vi "PowerControlDlg.vi"(3 "电源频率(Hz)":string="1", 8 "error out":errorcluster caption="error in") -> (0 "error out":errorcluster, 1 "倍数":string, 2 "NY":bool, 4 "电源电压(V)out":string="1", 5 "电压系数out":string="10")   [LabVIEW 2014, in "PowerControl.lvlib"]
uses:
  PowerControl.lvlib
  Acquisition/HW Configuration.ctl
  DataBase/DataBase.lvlib
  DetectElecrodes/DetectElectros.lvlib
  Acquisition/Acquisitions.lvlib
panel:
  out "电流值":dbl
  in  "电流系数":string="10"
  in  "电压系数":string="0.01"
  in  "备注":string
  in  "退出":bool
  in  "退出按钮":bool
  in  "确定按钮":bool
  in  "电源电压(V)":string="1"
  # "（1V~5V）"
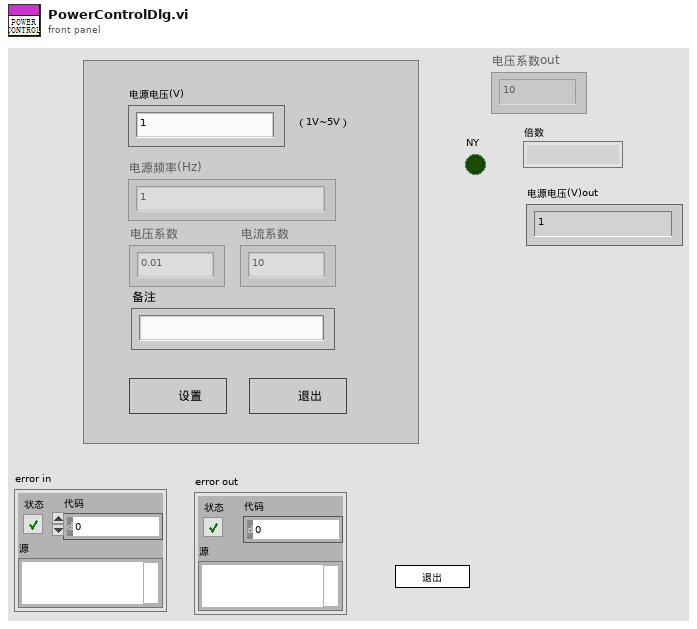
[diagram p1: front panel]
types:
  T1 = enum32{"invalid app kind", "Development System", "Run Time System", "Student Edition", "Embedded LabVIEW", "Evaluation", "Custom"}
  T2 = enum8{"Enabled", "Disabled", "Disabled and Grayed Out"}
  T3 = enum32{"Invalid", "Standard", "Closed", "Hidden", "Minimized", "Maximized"}
  T4 = typedef "Acquisitions.lvlib/HW Configuration.ctl" = cluster{"Physical Channel":tag, "Maximum Input":dbl, "Minimum Input":dbl, "Sample Rate":dbl, "Number of Samples":i32}
  T5 = cluster{"Core":cluster{"Current VI Reference":refnum<vi>, "Close Panel on Exit?":bool}, "Your Boolean data":bool, "Your string data":string, "V值":dbl, "倍数":string, "实际V值":string}
  T6 = cluster{"Current VI Reference":refnum<vi>, "Close Panel on Exit?":bool}
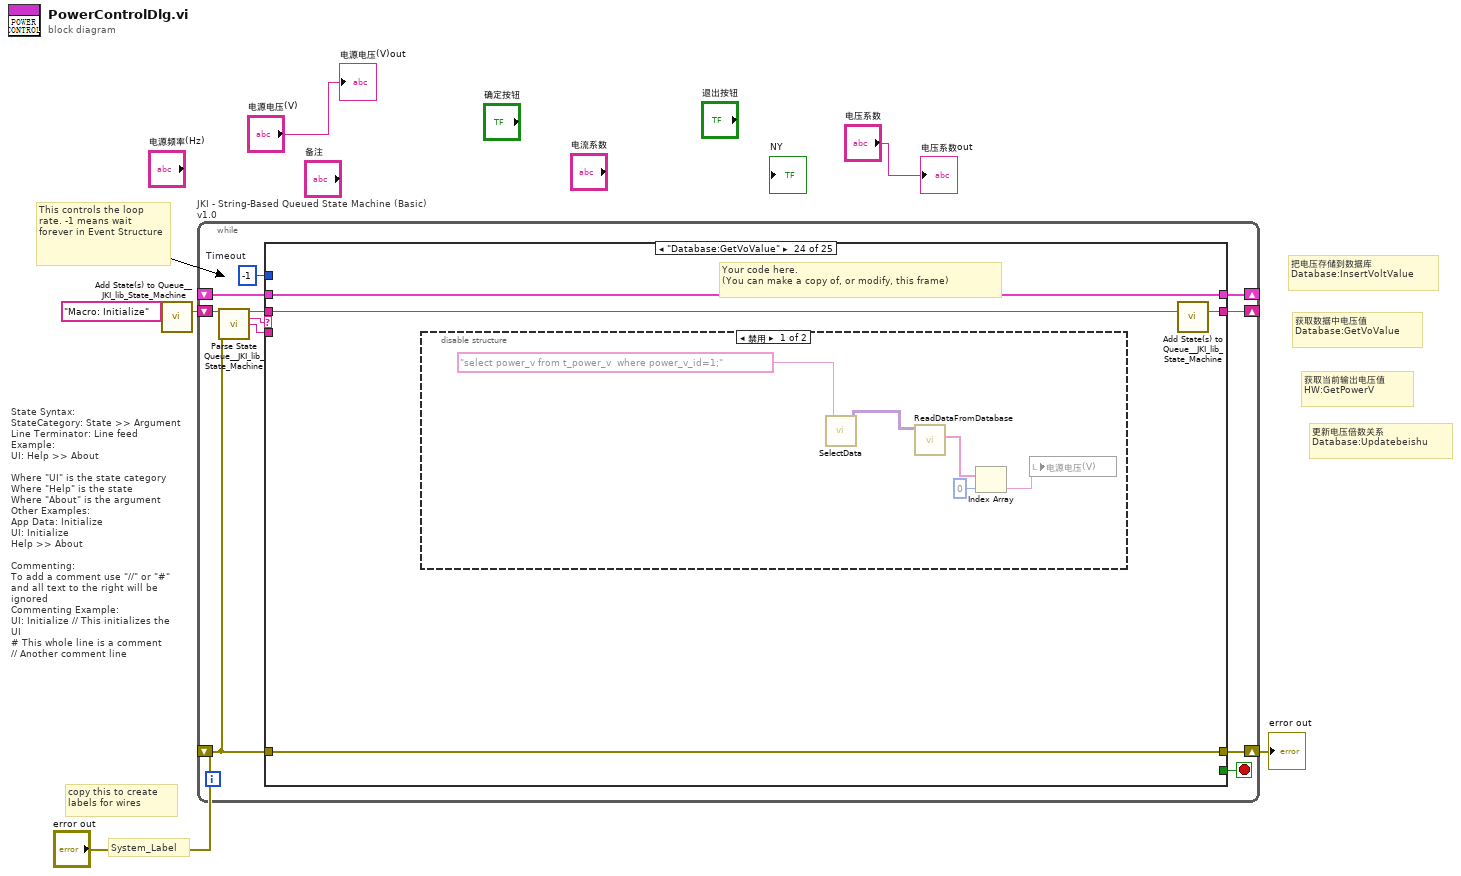
[diagram p0: block diagram]
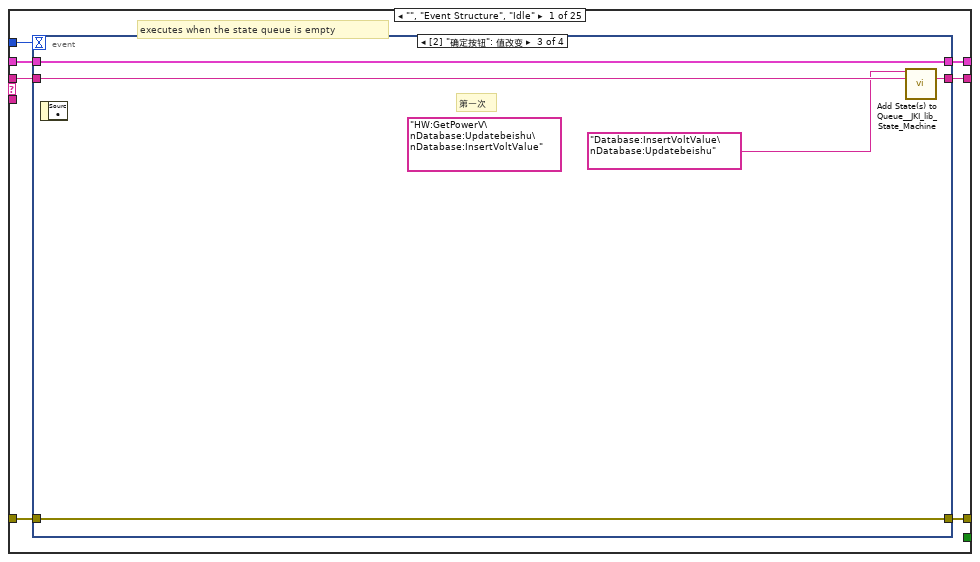
[diagram p2: hidden frame]
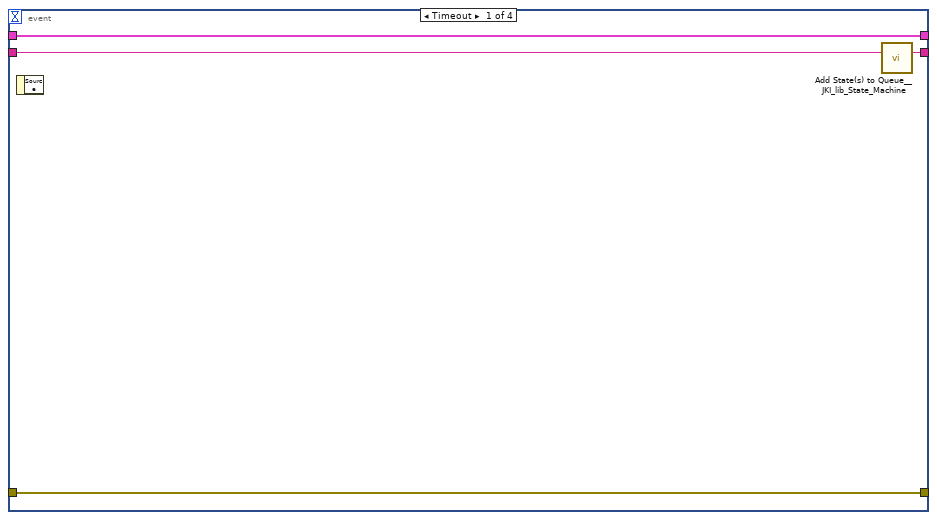
[diagram p3: hidden frame]
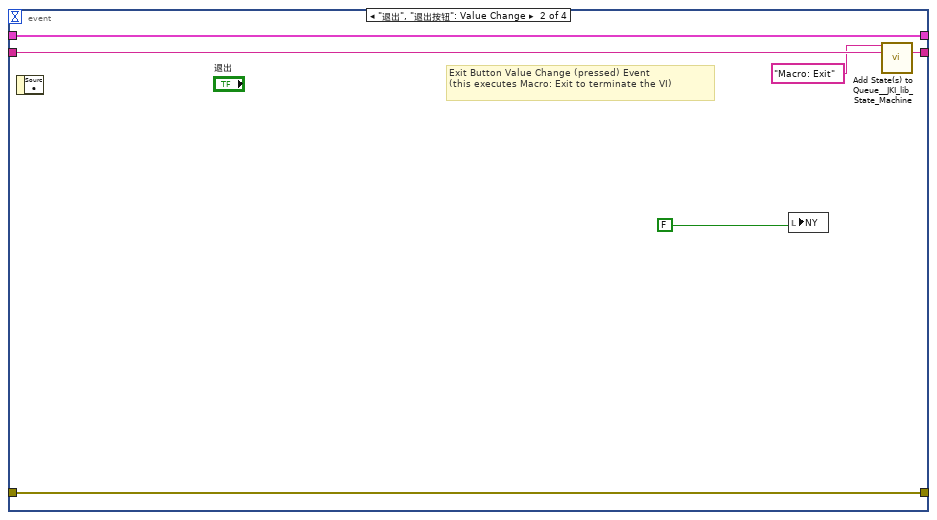
[diagram p4: hidden frame]
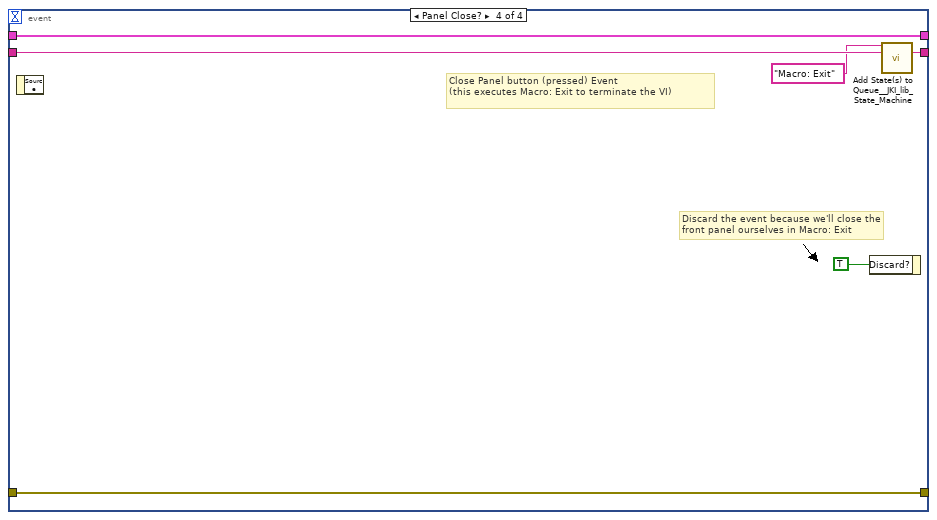
[diagram p5: hidden frame]
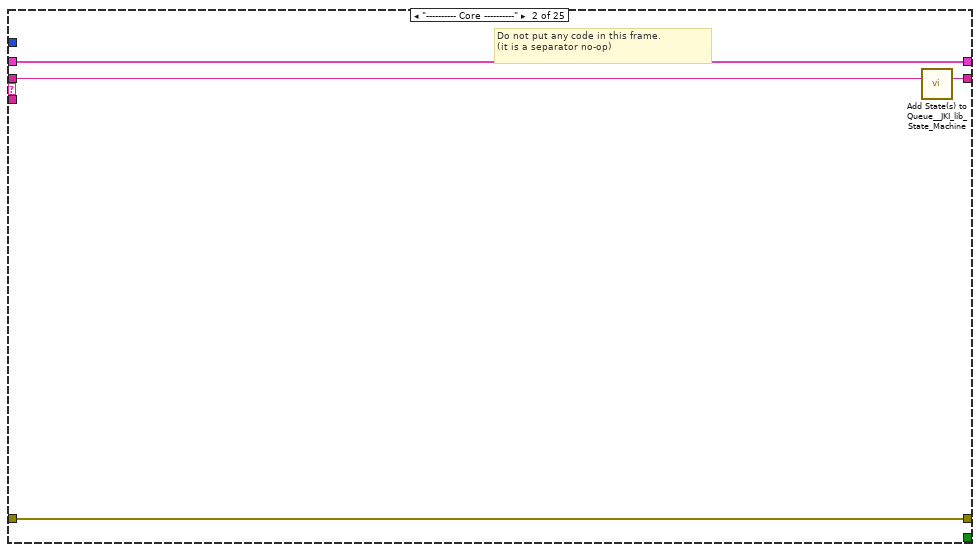
[diagram p6: hidden frame]
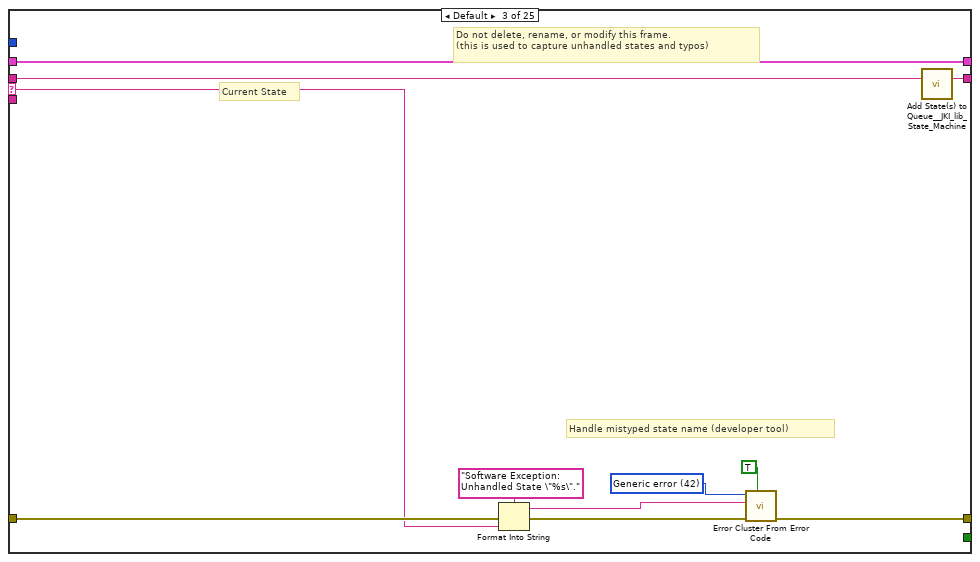
[diagram p7: hidden frame]
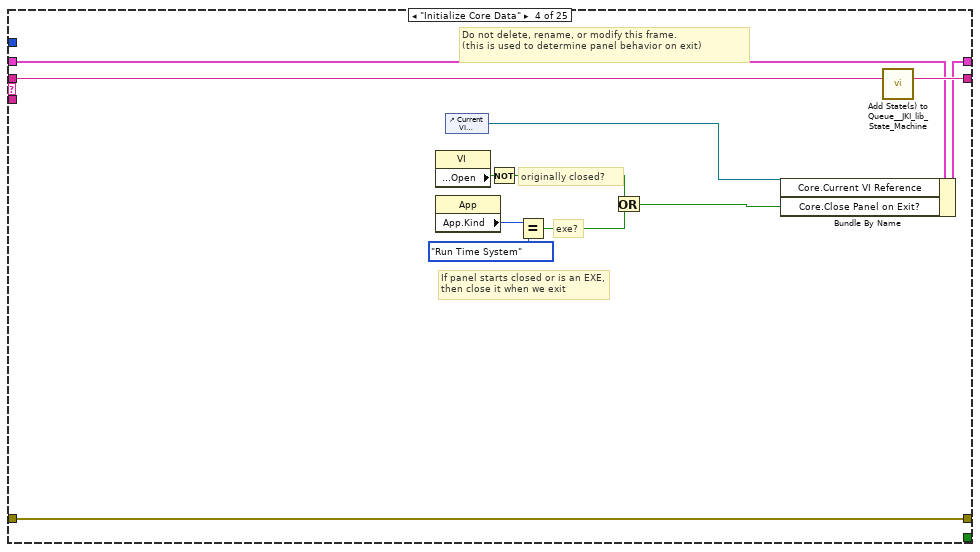
[diagram p8: hidden frame]
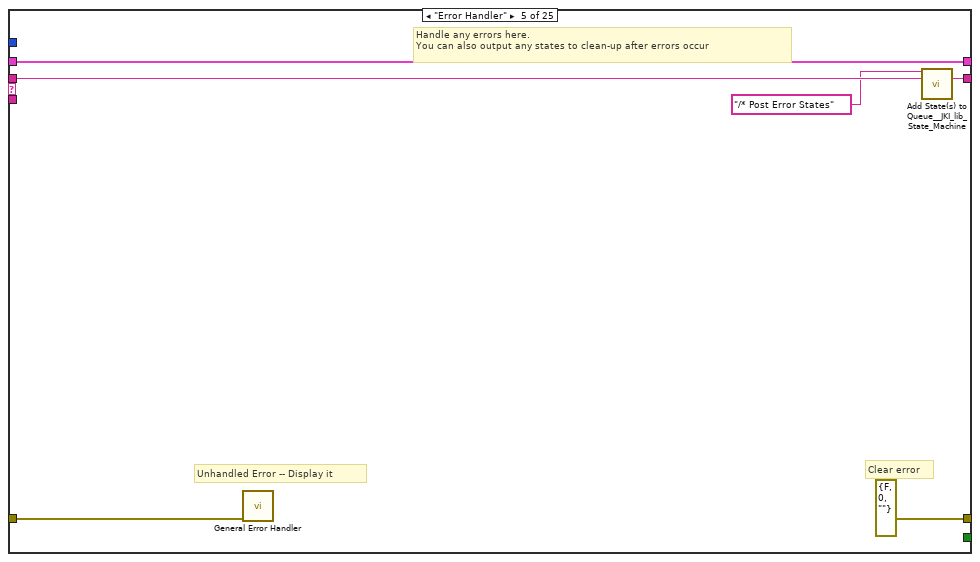
[diagram p9: hidden frame]
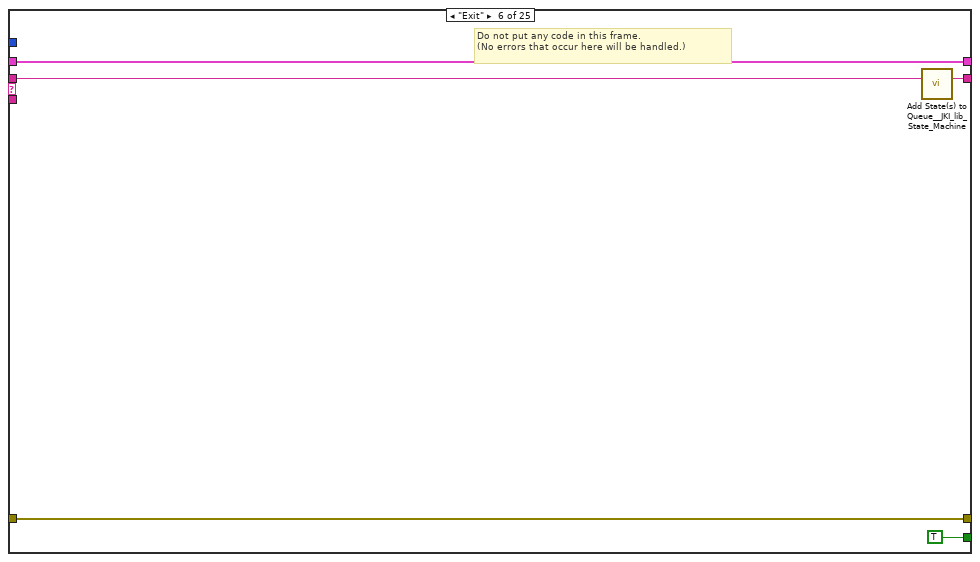
[diagram p10: hidden frame]
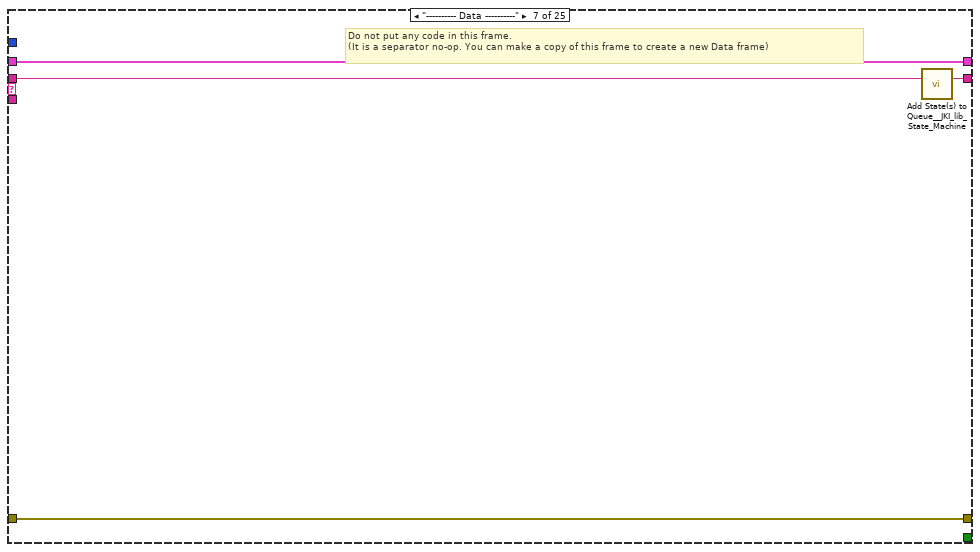
[diagram p11: hidden frame]
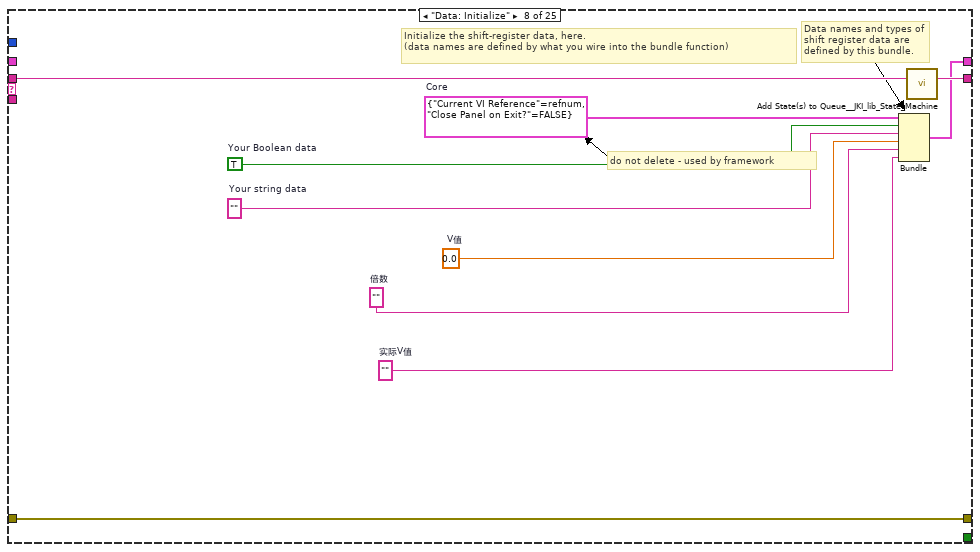
[diagram p12: hidden frame]
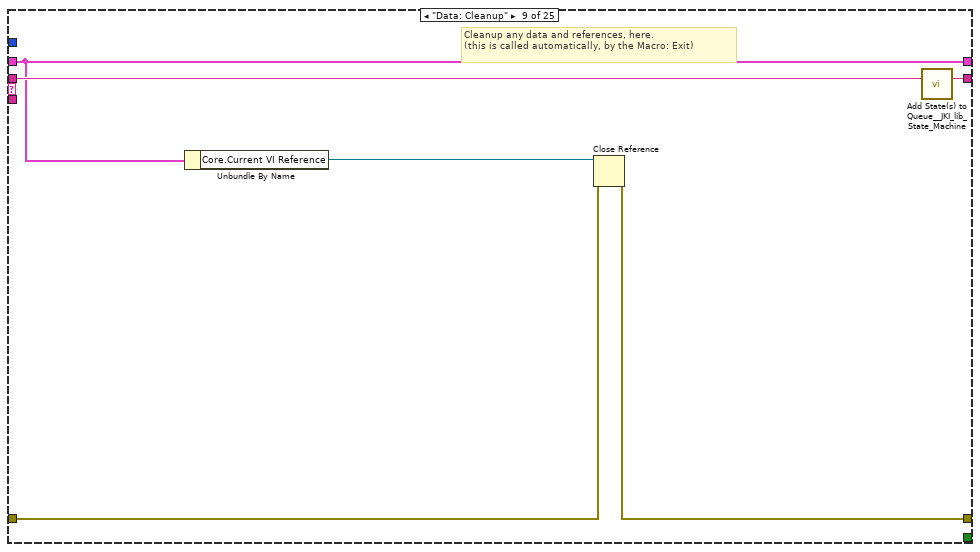
[diagram p13: hidden frame]
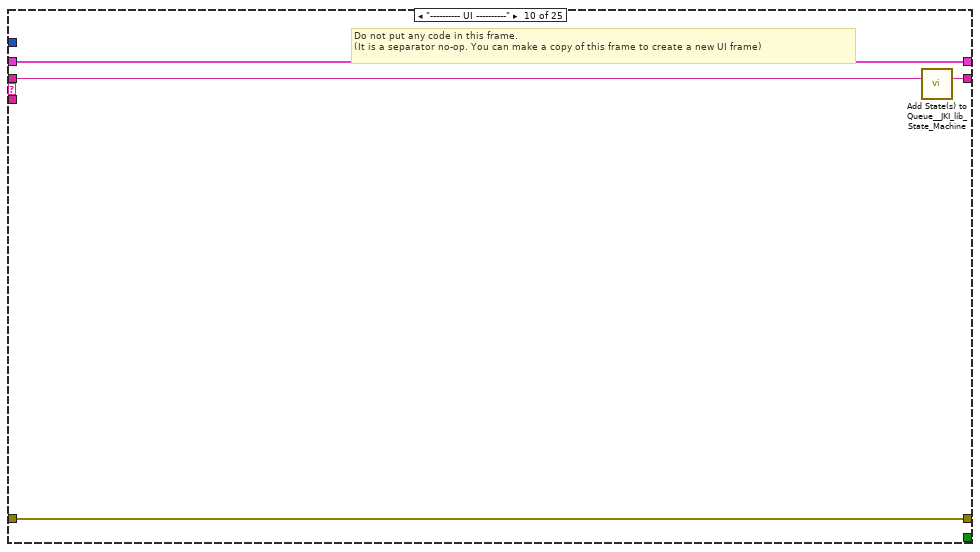
[diagram p14: hidden frame]
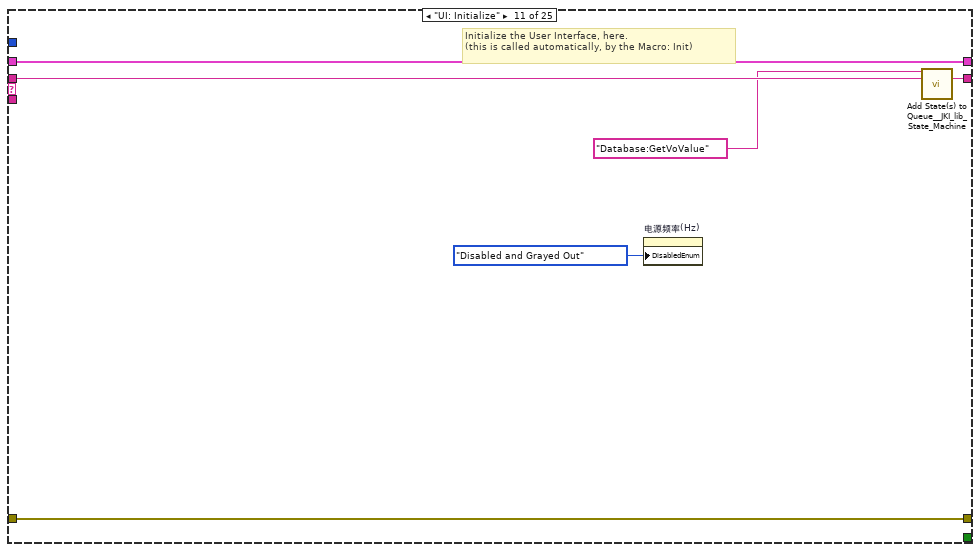
[diagram p15: hidden frame]
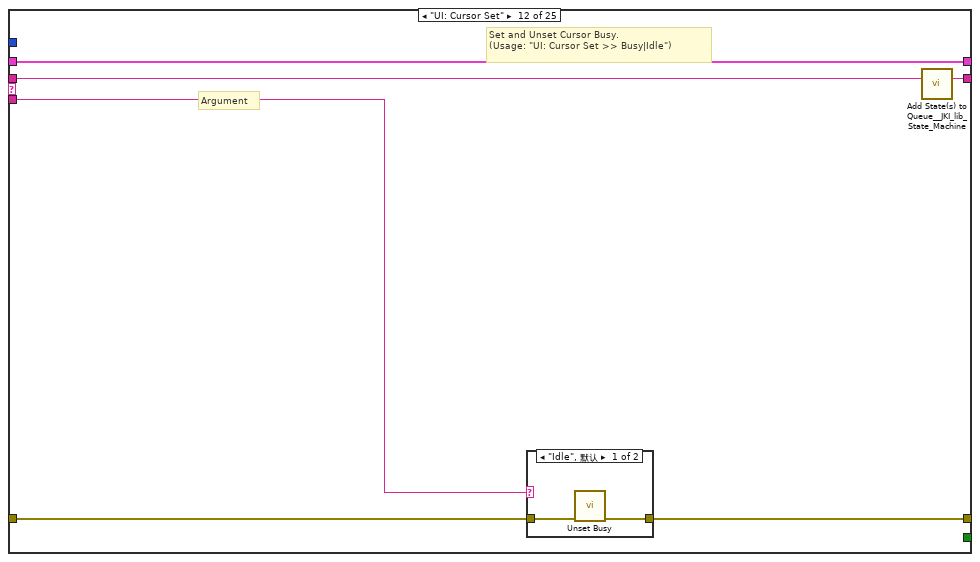
[diagram p16: hidden frame]
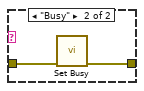
[diagram p17: hidden frame]
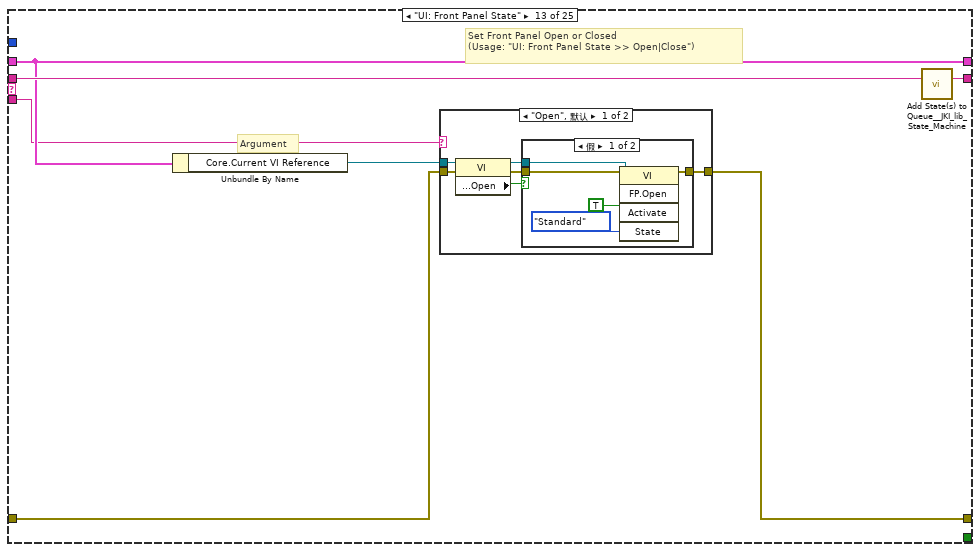
[diagram p18: hidden frame]
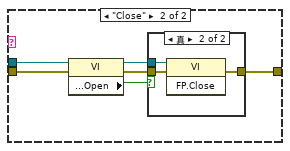
[diagram p20: hidden frame]
diagram:
  # "更新电压倍数关系\nDatabase:Updatebeishu"
  # "获取当前输出电压值\nHW:GetPowerV"
  # "获取数据中电压值\nDatabase:GetVoValue"
  # "把电压存储到数据库\nDatabase:InsertVoltValue"
  # "State Syntax:\nStateCategory: State >> Argument\nLine Terminator: Line feed\nExample:\nUI: Help >> About\n\nWhere \"UI\" is the state category\nWhere \"Help\" is the state\nWhere \"About\" is the argument\nOther Examples:\nApp Data: Initialize\nUI: Initialize\nHelp >> About\n\nCommenting:\nTo add a comment use \"//\" or \"#\" and all text to the right will be ignored\nCommenting Example:\nUI: Initialize // This initializes the UI\n# This whole line is a comment\n// Another comment line"
  # "copy this to create labels for wires"
  # "This controls the loop rate. -1 means wait forever in Event Structure"
  # "System_Label"
  n1 = call <vilib>:"Add State(s) to Queue__JKI_lib_State_Machine.vi"("State(s) in (\"\")"="Macro: Initialize") -> ("States Out"=w6:string)  [unwired: 14 in]
  n2 = while "JKI - String-Based Queued State Machine (Basic) v1.0" {
    shift-right: [w10] -> _
    shift-left: _ -> [w9]
    shift-right: [w13] -> w3
    shift-left: "error out" -> [w7]
    shift-right: [w12] -> _
    shift-left: w6 -> [w14]
    stop <- w11 stop-if-true
    w8 = -1  # Timeout
    n3 = call <vilib>:"Parse State Queue__JKI_lib_State_Machine.vi"("State Queue"=w14, "Error In (no error)"=w7) -> ("Remaining States"=w16:string, "Current State"=w17:string, "Arguments"=w15:string)  [unwired: 11 in]
    n4 = case shown="\"Database:GetVoValue\"" w17 {
      selector: w17 -> [_ _ w50 _ _ _ _ _ _ _ _ _ _ _ _ _ _ _ _ _ _ _ _ _ _]
      tunnel: w16 -> [w24 w49 w54 w72 w78 w83 w87 w97 w103 w107 w113 w119 w130 w156 w161 w171 w175 w179 w183 w187 w212 w216 w224 w239 w253]
      tunnel: w15 -> [_ _ _ _ _ _ _ _ _ _ _ w114 w124 _ _ _ _ _ _ _ _ _ _ _ _]
      tunnel: w9 -> [w22 w46 w52 w63 w75 w81 w84 _ w98 w104 w111 w117 w126 w153 w158 w168 w172 w176 w180 w184 w209 w213 w221 w236 w250]
      tunnel: [w21 w47 w56 w69 errorcluster {"status"=FALSE, "code"=0, "source"=""} ("error out") w80 w85 w94 w99 w105 w110 w115 w127 w154 w159 w169 w173 w177 w181 w185 w210 w214 w222 w237 w251] -> w13
      tunnel: w7 -> [w20 w47 w55 w69 w74 w80 w85 w94 w100 w105 w110 w116 w128 w154 w159 w169 w173 w177 w181 w185 w210 w214 w222 w237 w251]
      tunnel: [w23 w48 w53 w71 w77 w82 w86 w96 w102 w106 w112 w118 w129 w155 w160 w170 w174 w178 w182 w186 w211 w215 w223 w238 w252] -> w12
      tunnel: [_ _ _ _ _ TRUE _ _ _ _ _ _ _ _ _ _ _ _ _ _ _ _ _ _ _] -> w11
      tunnel: [w19 w46 w52 w70 w75 w81 w84 w95 w98 w104 w111 w117 w126 w153 w158 w168 w172 w176 w180 w184 w208 w213 w221 w236 w250] -> w10
      tunnel: w8 -> [w18 _ _ _ _ _ _ _ _ _ _ _ _ _ _ _ _ _ _ _ _ _ _ _ _]
      frame "", "Event Structure", "Idle" {
        # "executes when the state queue is empty"
        n5 = event shown="[2] \"确定按钮\": 值改变" {
          selector: _ -> [_ _ _ _]
          dyn-events: _ -> [_ _ _ _]
          timeout: w18 -> [_ _ _ _]
          tunnel: w24 -> [w28 w34 w39 w45]
          tunnel: [w27 w33 w38 w44] -> w23
          tunnel: w22 -> [w25 w31 w36 w42]
          tunnel: [w26 w32 w37 w43] -> w21
          tunnel: w20 -> [w26 w32 w37 w43]
          tunnel: [w25 w31 w36 w42] -> w19
          event Timeout {
            n6 = event-data() -> ()  [unwired: 1 in, 1 out]
            n7 = call <vilib>:"Add State(s) to Queue__JKI_lib_State_Machine.vi"("State(s) in (\"\")"=w28) -> ("States Out"=w27:string)  [unwired: 14 in]
          }
          event "退出", "退出按钮": Value Change {
            # "Exit Button Value Change (pressed) Event\n(this executes Macro: Exit to terminate the VI)"
            n8 = event-data() -> ()  [unwired: 1 in, 1 out]
            n9 = local write "NY"(FALSE) -> ()
            n10 = call <vilib>:"Add State(s) to Queue__JKI_lib_State_Machine.vi"("State(s) in Front (\"\")"="Macro: Exit", "State(s) in (\"\")"=w34) -> ("States Out"=w33:string)  [unwired: 13 in]
          }
          event "确定按钮": Value Change {
            (unwired) "HW:GetPowerV\nDatabase:Updatebeishu\nDatabase:InsertVoltValue"
            # "第一次"
            n11 = event-data() -> ()  [unwired: 1 in, 1 out]
            n12 = call <vilib>:"Add State(s) to Queue__JKI_lib_State_Machine.vi"("State(s) in Front (\"\")"="Database:InsertVoltValue\nDatabase:Updatebeishu", "State(s) in (\"\")"=w39) -> ("States Out"=w38:string)  [unwired: 13 in]
          }
          event Panel Close? {
            # "Discard the event because we'll close the front panel ourselves in Macro: Exit"
            # "Close Panel button (pressed) Event\n(this executes Macro: Exit to terminate the VI)"
            n13 = event-data() -> ()  [unwired: 1 in, 1 out]
            n14 = event-data("Discard?"=TRUE) -> ()  [unwired: 1 in, 1 out]
            n15 = call <vilib>:"Add State(s) to Queue__JKI_lib_State_Machine.vi"("State(s) in Front (\"\")"="Macro: Exit", "State(s) in (\"\")"=w45) -> ("States Out"=w44:string)  [unwired: 13 in]
          }
        }
      }
      frame "---------- Core ----------" {
        # "Do not put any code in this frame.\n(it is a separator no-op)"
        n16 = call <vilib>:"Add State(s) to Queue__JKI_lib_State_Machine.vi"("State(s) in (\"\")"=w49) -> ("States Out"=w48:string)  [unwired: 14 in]
      }
      frame Default {
        w59 = 42 items=["No error", "Argument error", "Memory is full", "Out of zone", "End of file", "File already open", "Generic file I/O error", "File not found", "File permission error", "Disk is full", "Duplicate path", "Too many files open", "System feature not enabled", "Resource file not found", "Cannot add resource", "Resource not found", "Image not found", "Image memory error", "Pen does not exist", "Config type invalid", "Config token not found", "Config parse error", "Config memory error", "Bad external code format", "Bad external code offset", "External code not present", "Null window", "Destroy window error", "Null menu", "Print aborted", "Bad print record", "Print driver error", "Windows error during printing", "Memory error during printing", "Print dialog error", "Generic print error", "Invalid device refnum", "Device not found", "Device parameter error", "Device unit error", "Cannot open device", "Device call aborted", "Generic error", "Cancelled by user", "Object ID too low", "Object ID too high", "Object not in heap", "Unknown heap", "Unknown object (invalid DefProc)", "Unknown object (DefProc not in table)", "Message out of range", "Invalid (null) method", "Unknown message", "Manager call not supported", "Bad address", "Network operation in progress", "Network operation timed out", "Connection is busy", "Network attribute not supported", "Network error", "Address in use", "System out of memory", "Connection aborted", "Connection refused", "Not connected", "Already connected", "Connection closed", "Initialization error (interapplication manager)", "Bad occurrence", "Wait on unbound occurrence handler", "Occurrence queue overflow", "Datalog type conflict", "Unused", "Unrecognized type (interapplication manager)", "Memory corrupt", "Failed to make temporary DLL", "Old CIN version", "Drag socket not found", "Failed to load drop-object", "Failed to register OLE object", "Failed to release OLE object", "Format specifier type mismatch", "Unknown format specifier", "Too few format specifiers", "Too many format specifiers", "Scan failed", "Newer CIN version", "Error converting to variant", "Runtime menu error", "Password tampered", "Variant attribute not found", "Incompatible variant data type", "Event data is not available", "Event Store is not present", "Occurrence is not found", "Event Queue is not created", "Event info is not available", "Refnum passed is NULL", "Error retrieving Class GUID", "Error retrieving CoClass GUID", "Error retrieving TypeLib GUID.", "Bad built application magic bytes.", "Specific driver is different from the specific driver associated with the Logical Name.", "There is no session opened to the class driver.", "Max Error", "MAX - Error with config objects", "MAX - Error loading configuration", "MAX - Group not supported"]
        # "Current State"
        # "Do not delete, rename, or modify this frame.\n(this is used to capture unhandled states and typos)"
        # "Handle mistyped state name (developer tool)"
        n17 = Format Into String(format string="Software Exception: Unhandled State \"%s\"." ("message"), error in=w55, w50) -> (resulting string=w58:string, error out=w57:errorcluster)  [unwired: 1 in]
        n18 = call <vilib>:"Error Cluster From Error Code.vi"("show call chain? (False)"=TRUE, "error in (no error)"=w57, "error message (\"\")"=w58, "error code (0)"=w59) -> ("error out"=w56:errorcluster)  [unwired: 5 in]
        n19 = call <vilib>:"Add State(s) to Queue__JKI_lib_State_Machine.vi"("State(s) in (\"\")"=w54) -> ("States Out"=w53:string)  [unwired: 14 in]
      }
      frame "Initialize Core Data" {
        # "Do not delete, rename, or modify this frame.\n(this is used to determine panel behavior on exit)"
        # "originally closed?"
        # "exe?"
        # "If panel starts closed or is an EXE, then close it when we exit"
        n20 = property class="VI"() -> ("Front Panel.Open"=w68:bool)  [unwired: 2 in, 2 out]
        n21 = property class="App"() -> ("App.Kind"=w67:T1)  [unwired: 2 in, 2 out]
        n22 = control-ref of="Current VI Reference"() -> (w61:refnum<vi>)
        n23 = Not(x=w68) -> (.not. x?=w65:bool)
        n24 = Equal?(x=w67, y=T1."Run Time System" ("Application:Kind")) -> (x = y?=w64:bool)
        n25 = Or(x=w65, y=w64) -> (x .or. y?=w62:bool)
        n26 = Bundle By Name(cluster=w63, "Core.Current VI Reference"=w61, "Core.Close Panel on Exit?"=w62) -> (w70:T5)
        n27 = call <vilib>:"Add State(s) to Queue__JKI_lib_State_Machine.vi"("State(s) in (\"\")"=w72) -> ("States Out"=w71:string)  [unwired: 14 in]
      }
      frame "Error Handler" {
        # "Unhandled Error -- Display it"
        # "Handle any errors here.\nYou can also output any states to clean-up after errors occur"
        # "Clear error"
        n28 = call <vilib>:"General Error Handler.vi"("error in (no error)"=w74) -> ()  [unwired: 10 in, 5 out]
        n29 = call <vilib>:"Add State(s) to Queue__JKI_lib_State_Machine.vi"("State(s) in Front (\"\")"="/* Post Error States", "State(s) in (\"\")"=w78) -> ("States Out"=w77:string)  [unwired: 13 in]
      }
      frame "Exit" {
        # "Do not put any code in this frame.\n(No errors that occur here will be handled.)"
        n30 = call <vilib>:"Add State(s) to Queue__JKI_lib_State_Machine.vi"("State(s) in (\"\")"=w83) -> ("States Out"=w82:string)  [unwired: 14 in]
      }
      frame "---------- Data ----------" {
        # "Do not put any code in this frame.\n(It is a separator no-op. You can make a copy of this frame to create a new Data frame)"
        n31 = call <vilib>:"Add State(s) to Queue__JKI_lib_State_Machine.vi"("State(s) in (\"\")"=w87) -> ("States Out"=w86:string)  [unwired: 14 in]
      }
      frame "Data: Initialize" {
        w88 = ""  # 实际V值
        w89 = ""  # 倍数
        w90 = 0.0  # V值
        w91 = T6 {"Current VI Reference"=refnum, "Close Panel on Exit?"=FALSE}  # Core
        w93 = TRUE  # Your Boolean data
        w92 = ""  # Your string data
        # "do not delete - used by framework"
        # "Data names and types of shift register data are defined by this bundle."
        # "Initialize the shift-register data, here.\n(data names are defined by what you wire into the bundle function)"
        n32 = Bundle("Core"=w91, "Your Boolean data"=w93, "Your string data"=w92, "V值"=w90, "倍数"=w89, "实际V值"=w88) -> (w95:T5)  [unwired: 1 in]
        n33 = call <vilib>:"Add State(s) to Queue__JKI_lib_State_Machine.vi"("State(s) in (\"\")"=w97) -> ("States Out"=w96:string)  [unwired: 14 in]
      }
      frame "Data: Cleanup" {
        # "Cleanup any data and references, here.\n(this is called automatically, by the Macro: Exit)"
        n34 = Unbundle By Name(w98) -> ("Core.Current VI Reference"=w101:refnum<vi>)
        n35 = Close Reference(reference=w101, error in (no error)=w100) -> (error out=w99:errorcluster)
        n36 = call <vilib>:"Add State(s) to Queue__JKI_lib_State_Machine.vi"("State(s) in (\"\")"=w103) -> ("States Out"=w102:string)  [unwired: 14 in]
      }
      frame "---------- UI ----------" {
        # "Do not put any code in this frame.\n(It is a separator no-op. You can make a copy of this frame to create a new UI frame)"
        n37 = call <vilib>:"Add State(s) to Queue__JKI_lib_State_Machine.vi"("State(s) in (\"\")"=w107) -> ("States Out"=w106:string)  [unwired: 14 in]
      }
      frame "UI: Initialize" {
        # "Initialize the User Interface, here.\n(this is called automatically, by the Macro: Init)"
        n38 = property on="电源频率(Hz)" class="Str"("DisabledEnum"=T2."Disabled and Grayed Out" ("禁用")) -> ()  [unwired: 2 in, 2 out]
        n39 = call <vilib>:"Add State(s) to Queue__JKI_lib_State_Machine.vi"("State(s) in Front (\"\")"="Database:GetVoValue", "State(s) in (\"\")"=w113) -> ("States Out"=w112:string)  [unwired: 13 in]
      }
      frame "UI: Cursor Set" {
        # "Argument"
        # "Set and Unset Cursor Busy.\n(Usage: \"UI: Cursor Set >> Busy|Idle\")"
        n40 = case shown="\"Idle\", 默认" w114 {
          tunnel: w116 -> [w121 w123]
          tunnel: [w120 w122] -> w115
          frame "Idle", Default {
            n41 = call <vilib>:"Unset Busy.vi"("error in (no error)"=w121) -> ("error out"=w120:errorcluster)  [unwired: 10 in]
          }
          frame "Busy" {
            n42 = call <vilib>:"Set Busy.vi"("error in (no error)"=w123) -> ("error out"=w122:errorcluster)  [unwired: 9 in, 1 out]
          }
        }
        n43 = call <vilib>:"Add State(s) to Queue__JKI_lib_State_Machine.vi"("State(s) in (\"\")"=w119) -> ("States Out"=w118:string)  [unwired: 14 in]
      }
      frame "UI: Front Panel State" {
        # "Argument"
        # "Set Front Panel Open or Closed\n(Usage: \"UI: Front Panel State >> Open|Close\")"
        n44 = Unbundle By Name(w126) -> ("Core.Current VI Reference"=w125:refnum<vi>)
        n45 = case shown="\"Open\", 默认" w124 {
          tunnel: w128 -> [w134 w147]
          tunnel: [w136 w148] -> w127
          tunnel: w125 -> [w135 w145]
          frame "Open", Default {
            n46 = property class="VI"(reference=w135, error in=w134) -> (reference out=w132:refnum<vi>, error out=w133:errorcluster, "Front Panel.Open"=w131:bool)
            n47 = case shown="假" w131 {
              tunnel: [w139 w142] -> w136
              tunnel: w133 -> [w138 w142]
              tunnel: w132 -> [w137 _]
              frame False {
                n48 = invoke class="VI" method="FP.Open"(reference=w137, error in=w138, "Activate"=TRUE, "State"=T3."Standard") -> (error out=w139:errorcluster)  [unwired: 1 in, 4 out]
              }
              frame True {
              }
            }
          }
          frame "Close" {
            n49 = property class="VI"(reference=w145, error in=w147) -> (reference out=w144:refnum<vi>, error out=w146:errorcluster, "Front Panel.Open"=w143:bool)
            n50 = case shown="真" w143 {
              tunnel: [w149 w152] -> w148
              tunnel: w146 -> [w149 w151]
              tunnel: w144 -> [_ w150]
              frame False {
              }
              frame True {
                n51 = invoke class="VI" method="FP.Close"(reference=w150, error in=w151) -> (error out=w152:errorcluster)  [unwired: 1 in, 2 out]
              }
            }
          }
        }
        n52 = call <vilib>:"Add State(s) to Queue__JKI_lib_State_Machine.vi"("State(s) in (\"\")"=w130) -> ("States Out"=w129:string)  [unwired: 14 in]
      }
      frame "---------- Macro ----------" {
        # "Do not put any code in this frame.\n(It is a separator no-op. You can make a copy of this frame to create a new Macro frame)"
        n53 = call <vilib>:"Add State(s) to Queue__JKI_lib_State_Machine.vi"("State(s) in (\"\")"=w156) -> ("States Out"=w155:string)  [unwired: 14 in]
      }
      frame "Macro: Initialize" {
        w157 = "Data: Initialize\nInitialize Core Data\nUI: Initialize\nUI: Front Panel State >> Open"  # Data: Initialize Initialize Core Data UI: Initialize UI: Front Panel State >> Open
        # "Initialization Macro\n(This is called once, when the VI starts)"
        n54 = call <vilib>:"Add State(s) to Queue__JKI_lib_State_Machine.vi"("State(s) in Front (\"\")"=w157, "State(s) in (\"\")"=w161) -> ("States Out"=w160:string)  [unwired: 13 in]
      }
      frame "Macro: Exit" {
        # "Exit Macro\n(This is called once, when the VI exits)"
        n55 = Unbundle By Name(w168) -> ("Core.Close Panel on Exit?"=w167:bool)
        n56 = Select(t="UI: Front Panel State >> Close", s=w167, f="") -> (s? t:f=w164:string)
        n57 = call <vilib>:"Add State(s) to Queue__JKI_lib_State_Machine.vi"("State(s) in (\"\")"=w164, "State(s) at Back (\"\")"="Data: Cleanup\nExit") -> ("States Out"=w162:string)  [unwired: 13 in]
        n58 = call <vilib>:"Add State(s) to Queue__JKI_lib_State_Machine.vi"("State(s) in Front (\"\")"=w162, "State(s) in (\"\")"=w171) -> ("States Out"=w170:string)  [unwired: 13 in]
      }
      frame "---------- New Category ----------" {
        # "Template Separator\n(You can make a copy of, or modify, this frame)"
        n59 = call <vilib>:"Add State(s) to Queue__JKI_lib_State_Machine.vi"("State(s) in (\"\")"=w175) -> ("States Out"=w174:string)  [unwired: 14 in]
      }
      frame "New Category: 1" {
        # "Your code here.\n(You can make a copy of, or modify, this frame)"
        n60 = call <vilib>:"Add State(s) to Queue__JKI_lib_State_Machine.vi"("State(s) in (\"\")"=w179) -> ("States Out"=w178:string)  [unwired: 14 in]
      }
      frame "New Category: 2" {
        # "Your code here.\n(You can make a copy of, or modify, this frame)"
        n61 = call <vilib>:"Add State(s) to Queue__JKI_lib_State_Machine.vi"("State(s) in (\"\")"=w183) -> ("States Out"=w182:string)  [unwired: 14 in]
      }
      frame "---------HW--------" {
        # "Your code here.\n(You can make a copy of, or modify, this frame)"
        n62 = call <vilib>:"Add State(s) to Queue__JKI_lib_State_Machine.vi"("State(s) in (\"\")"=w187) -> ("States Out"=w186:string)  [unwired: 14 in]
      }
      frame "HW:GetPowerV" {
        # "求现在电源倍数关系40*getV/setV"
        # "Your code here.\n(You can make a copy of, or modify, this frame)"
        n63 = local read "电源电压(V)"() -> (w207:string)
        n64 = Fract/Exp String To Number(string=w207) -> (number=w188:dbl)  [unwired: 3 in, 1 out]
        n65 = local read "电压系数"() -> (w196:string)
        n66 = call "AcquireVandA.vi"("Hardware Configuration"=T4 {"Physical Channel"="Dev18/ai0", "Maximum Input"=10.0, "Minimum Input"=-10.0, "Sample Rate"=5000.0, "Number of Samples"=5000}) -> ("Graph Data"=w204:waveform(dbl)[])  [unwired: 8 in, 1 out]
        n67 = local read "电源频率(Hz)"() -> (w202:string)
        n68 = Split Signals(w204) -> (w206:dynamicdata, w194:dynamicdata)  [unwired: 2 in]
        n69 = Fract/Exp String To Number(string=w196) -> (number=w195:dbl)  [unwired: 3 in, 1 out]
        n70 = Decimal String To Number(string=w202) -> (number=w193:i32)  [unwired: 2 in, 1 out]
        n71 = call "从动态数据转换2"("Dynamic Data Type"=w194) -> ("Array"=w192:dbl[])  [unwired: 3 in]
        n72 = call "从动态数据转换"("Dynamic Data Type"=w206) -> ("Array"=w203:dbl[])  [unwired: 3 in]
        n73 = call "1chFFT.vi"("Array"=w192, "频率"=w193) -> ("幅度值"=w191:dbl)  [unwired: 2 in, 1 out]
        n74 = call "1chFFT.vi"("Array"=w203, "频率"=w193) -> ("幅度值"=w201:dbl)  [unwired: 2 in, 1 out]
        n75 = Divide(x=w201, y=w188) -> (x/y=w197:dbl)
        n76 = Divide(x=w191, y=5.0) -> (x/y=→"电流值":dbl)
        n77 = Divide(x=w197, y=w195) -> (x/y=w198:dbl)
        n78 = Number To Fractional String(number=w201) -> (F-format string=w200:string)  [unwired: 3 in]
        n79 = Number To Fractional String(number=w198) -> (F-format string=w199:string)  [unwired: 3 in]
        n80 = Bundle By Name(cluster=w209, "V值"=w201, "倍数"=w199, "实际V值"=w200) -> (w208:T5)
        n81 = call <vilib>:"Add State(s) to Queue__JKI_lib_State_Machine.vi"("State(s) in (\"\")"=w212) -> ("States Out"=w211:string)  [unwired: 14 in]
      }
      frame "-----------Database---------" {
        # "Your code here.\n(You can make a copy of, or modify, this frame)"
        n82 = call <vilib>:"Add State(s) to Queue__JKI_lib_State_Machine.vi"("State(s) in (\"\")"=w216) -> ("States Out"=w215:string)  [unwired: 14 in]
      }
      frame "Database:Updatebeishu" {
        # "Your code here.\n(You can make a copy of, or modify, this frame)"
        n83 = flat-sequence {
          tunnel: w220 -> [w227]
          tunnel: [w226] -> w219
          tunnel: w218 -> [w225]
          tunnel: w219 -> [_]
          tunnel: ["Macro: Exit"] -> w217
          frame #0 {
            n84 = disable-structure shown="禁用" {
              disable-tunnel: w227 -> [w230 _]
              disable-tunnel: [w229 _] -> w226
              disable-tunnel: w225 -> [w228 _]
              frame Disabled {
                n85 = Format Into String(format string="update t_power_v set power_beishu='%s',\npower_shiji_v='%s' where power_v_id=1;", w230, w228) -> (resulting string=w232:string)  [unwired: 2 in, 1 out]
                n86 = call "updateData.vi"("SQL query"=w232) -> ("error out"=w229:errorcluster)  [unwired: 10 in]
              }
              frame Enabled {
              }
            }
          }
          frame #1 {
            n87 = One Button Dialog(message="设置成功" ("消息")) -> ()  [unwired: 1 in, 1 out]
            n88 = local write "NY"(TRUE) -> ()
          }
        }
        n89 = Unbundle By Name(w221) -> ("倍数"=w220:string, "实际V值"=w218:string)
        "倍数" <- w220
        n90 = call <vilib>:"Add State(s) to Queue__JKI_lib_State_Machine.vi"("State(s) in Front (\"\")"=w217, "State(s) in (\"\")"=w224) -> ("States Out"=w223:string)  [unwired: 13 in]
      }
      frame "Database:GetVoValue" {
        # "Your code here.\n(You can make a copy of, or modify, this frame)"
        n91 = disable-structure shown="禁用" {
          frame Disabled {
            n92 = call "SelectData.vi"("SQL query"="select power_v from t_power_v  where power_v_id=1;") -> ("recordset data"=w243:variant[][])  [unwired: 7 in, 1 out]
            n93 = call "ReadDataFromDatabase.vi"("recordset data"=w243) -> ("一行记录"=w242:string[])  [unwired: 9 in, 1 out]
            n94 = Index Array(array=w242, index=0 ("索引")) -> (element=w240:string)
            n95 = local write "电源电压(V)"(w240) -> ()
          }
          frame Enabled {
          }
        }
        n96 = call <vilib>:"Add State(s) to Queue__JKI_lib_State_Machine.vi"("State(s) in (\"\")"=w239) -> ("States Out"=w238:string)  [unwired: 14 in]
      }
      frame "Database:InsertVoltValue" {
        # "Your code here.\n(You can make a copy of, or modify, this frame)"
        n97 = local read "电源频率(Hz)"() -> (w246:string)
        n98 = local read "电源电压(V)"() -> (w248:string)
        n99 = local read "备注"() -> (w245:string)
        n100 = Format Into String(format string="update t_power_v set\npower_v='%s',power_f='%s',power_v_desc='%s'\nwhere power_v_id=1;", w248, w246, w245) -> (resulting string=w247:string)  [unwired: 2 in, 1 out]
        n101 = call "updateData.vi"("SQL query"=w247) -> ()  [unwired: 10 in, 1 out]
        n102 = call <vilib>:"Add State(s) to Queue__JKI_lib_State_Machine.vi"("State(s) in (\"\")"=w253) -> ("States Out"=w252:string)  [unwired: 14 in]
      }
    }
  }
  "error out" <- w3
  "电压系数out" <- "电压系数"
  "电源电压(V)out" <- "电源电压(V)"
